vi "_FPGA Set Digi Line.vi"(4 "error in":errorcluster, 5 "States":u16, 6 "Line (Set Latch1)":T1=enum."Set Latch1") -> (0 "error out":errorcluster)   [LabVIEW 2012]
uses:
  Type/_RW Status.ctl
  Type/_Pump Parameter.ctl
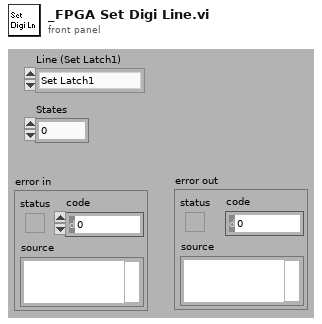
[diagram p1: front panel]
types:
  T1 = typedef "_RW Status.ctl" = enum8{"Done", "Do Read", "Do Write", "Set Latch1", "Set Latch2", "Set Latch3", "Set Latch4", "RP ON", "EL ON", "Serial Send", "Set LC Out", "Get LC In", "Read VAC", "Table Test", "Get Interlock", "Do Read2", "Do Write2"}
  T2 = typedef "_Pump Parameter.ctl" = enum16{"Turn Pump Motor On", "Turn Pump Motor Off", "Read Pump Oil Deficiency", "Read Rotation Switch Point Attained", "Read Ele. Drive Over Temperature", "Read Pump Over Temperature", "Read Set Rotation Speed Attained", "Read Turbopump Accelerates", "Read Actual Rotation Speed in Hz", "Read Motor Current in A", "Read Operating Hours in h", "Read Motor Voltage in V", "Read Motor Power in W", "Set Rotation Speed Switchpoint in %", "Clear Error", "Read Error Code", "Read Bearing Temperature", "Read Hardware Version", "Read Firmware Version", "Read Operating Hours (Drive)", "Read Rotational Speed (rpm)", "Read Power Stage Temperature", "Read Electronics Temperature", "Read Upper Pump Temperature", "Read Motor Temperature", "Read Error Code History, 1", "Read Error Code History, 2", "Read Error Code History, 3", "Read Error Code History, 4", "Read Error Code History, 5", "Read Error Code History, 6", "Read Error Code History, 7", "Read Error Code History, 8", "Read Error Code History, 9", "Read Error Code History, 10"}
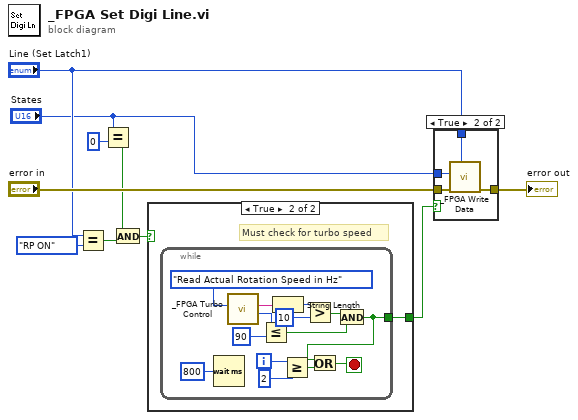
[diagram p0: block diagram]
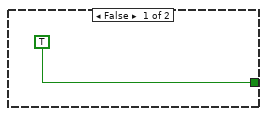
[diagram p3: hidden frame]
diagram:
  n1 = Equal?(x="Line (Set Latch1)", y=_RW_Status."RP ON") -> (x = y?=w4:bool)
  n2 = Equal?(x="States", y=u16 0) -> (x = y?=w1:bool)
  n3 = And(x=w1, y=w4) -> (x .and. y?=w3:bool)
  n4 = case shown="True" w3 {
    tunnel: [TRUE w12] -> w2
    frame False {
    }
    frame True {
      # "Must check for turbo speed"
      n5 = while {
        tunnel: [w14] -> w12
        i -> [w18]
        stop <- w13 stop-if-true
        n6 = Wait (ms)(milliseconds to wait=u32 800) -> ()  [unwired: 1 out]
        n7 = call "_FPGA Turbo Control.vi"("Command"=_Pump_Parameter."Read Actual Rotation Speed in Hz") -> ("Speed"=w24:i32, "Reply"=w23:string)  [unwired: 3 in, 4 out]
        n8 = Less Or Equal?(x=w24, y=90) -> (x <= y?=w19:bool)
        n9 = String Length(string=w23) -> (length=w21:i32)
        n10 = Greater Or Equal?(x=w18, y=2) -> (x >= y?=w15:bool)
        n11 = Greater?(x=w21, y=10) -> (0:w20:bool)
        n12 = And(x=w20, y=w19) -> (x .and. y?=w14:bool)
        n13 = Or(x=w14, y=w15) -> (x .or. y?=w13:bool)
      }
    }
  }
  n14 = case shown="True" w2 {
    tunnel: "error in" -> [w27 w31]
    tunnel: [w27 w30] -> w9
    tunnel: "Line (Set Latch1)" -> [_ w29]
    tunnel: "States" -> [_ w28]
    frame False {
    }
    frame True {
      n15 = call "_FPGA Write Data.vi"("Write Mode (Do Write)"=w29, "error in"=w31, "Address"=w28) -> ("error out"=w30:errorcluster)  [unwired: 3 in, 2 out]
    }
  }
  "error out" <- w9
